vi "Sender 12 new version.vi"   [LabVIEW 2012]
uses:
  <vilib>/NXT/Block Support/NXT_OutputPort.ctl
  <vilib>/NXT/Block Support/NXT_MessageMailbox.ctl
  <vilib>/NXT/Block Support/NXT_InputPort.ctl
  <vilib>/NXT/Dual Mode Library/Waits/Wait_Num.vi
  <vilib>/NXT/Dual Mode Library/Motors/Rotation.vi
  <vilib>/NXT/Dual Mode Library/Motors/ResetMotor.vi
  <vilib>/NXT/Dual Mode Library/BT/BlueTooth_Write_String.vi
  <vilib>/NXT/Dual Mode Library/Display/drawText.vi
types:
  T1 = typedef "LVHSConnector.ctl" = refnum<class "BrickReference.lvclass">
  T2 = typedef "NXT_InputPort.ctl" = u32
  T3 = typedef "NXT_MessageMailbox.ctl" = u8
  T4 = typedef "NXT_OutputPort.ctl" = u8
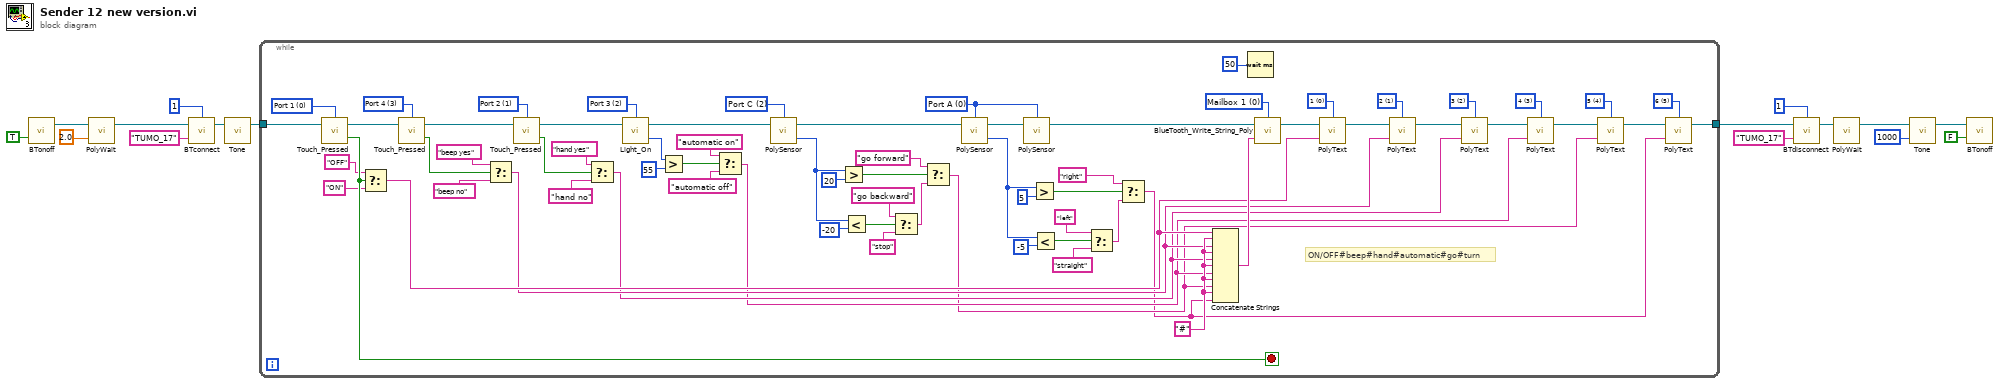
[diagram p0: block diagram]
diagram:
  n1 = call <vilib>:"BTonoff.vi"("On/Off"=TRUE) -> ("NXT/EV3"=w4:T1)  [unwired: 2 in, 1 out]
  n2 = call-poly <vilib>:"PolyWait.vi"("Time (1 sec)"=sgl 2.0, "NXT/EV3"=w4) -> ("NXT/EV3"=w3:T1)  [unwired: 2 in]
  n3 = call <vilib>:"BTconnect.vi"("Partner Name"="TUMO_17", "NXT/EV3"=w3, "Connection"=u8 1) -> ("NXT/EV3"=w10:T1)  [unwired: 1 out]
  n4 = call <vilib>:"Tone.vi"("NXT/EV3"=w10) -> ("NXT/EV3"=w9:T1)  [unwired: 3 in]
  n5 = while {
    tunnel: w9 -> [w67]
    tunnel: [w18] -> w1
    stop <- w66 stop-if-true
    w20 = i16 5 items=["1", "2", "3", "4", "5", "6", "7", "8", "9", "10", "11", "12"] ("Line")
    w23 = i16 4 items=["1", "2", "3", "4", "5", "6", "7", "8", "9", "10", "11", "12"] ("Line")
    w26 = i16 3 items=["1", "2", "3", "4", "5", "6", "7", "8", "9", "10", "11", "12"] ("Line")
    w29 = i16 2 items=["1", "2", "3", "4", "5", "6", "7", "8", "9", "10", "11", "12"] ("Line")
    w32 = i16 1 items=["1", "2", "3", "4", "5", "6", "7", "8", "9", "10", "11", "12"] ("Line")
    w34 = i16 0 items=["1", "2", "3", "4", "5", "6", "7", "8", "9", "10", "11", "12"] ("Line")
    w47 = T2 2 items=["Port 1", "Port 2", "Port 3", "Port 4"] ("Port (Port 1)")
    w55 = T2 1 items=["Port 1", "Port 2", "Port 3", "Port 4"] ("Port (Port 1)")
    w36 = "#" ("string")
    w69 = T2 0 items=["Port 1", "Port 2", "Port 3", "Port 4"] ("Port (Port 1)")
    w70 = u8 0 items=["Port A", "Port B", "Port C"] ("Port (Port A)")
    w78 = T2 3 items=["Port 1", "Port 2", "Port 3", "Port 4"] ("Port (Port 1)")
    w83 = T3 0 items=["Mailbox 1", "Mailbox 2", "Mailbox 3", "Mailbox 4", "Mailbox 5", "Mailbox 6", "Mailbox 7", "Mailbox 8", "Mailbox 9", "Mailbox 10"] ("Mailbox")
    w84 = T4 2 items=["Port A", "Port B", "Port C", "Port D"] ("Port (Port A)")
    # "ON/OFF#beep#hand#automatic#go#turn"
    n6 = call <vilib>:"Touch_Pressed.vi"("NXT/EV3"=w67, "Port (Port 1)"=w69) -> ("Yes / No"=w66:bool, "NXT/EV3"=w63:T1)  [unwired: 1 in]
    n7 = Select(t="OFF", s=w66, f="ON") -> (s? t:f=w33:string)
    n8 = call <vilib>:"Touch_Pressed.vi"("NXT/EV3"=w63, "Port (Port 1)"=w78) -> ("Yes / No"=w60:bool, "NXT/EV3"=w54:T1)  [unwired: 1 in]
    n9 = Select(t="beep yes", s=w60, f="beep no") -> (s? t:f=w30:string)
    n10 = call <vilib>:"Touch_Pressed.vi"("NXT/EV3"=w54, "Port (Port 1)"=w55) -> ("Yes / No"=w58:bool, "NXT/EV3"=w46:T1)  [unwired: 1 in]
    n11 = Select(t="hand yes", s=w58, f="hand no") -> (s? t:f=w27:string)
    n12 = call <vilib>:"Light_On.vi"("NXT/EV3"=w46, "Port (Port 3)"=w47) -> ("Scaled Value"=w45:i16, "NXT/EV3"=w42:T1)  [unwired: 1 in]
    n13 = Greater?(x=w45, y=i16 55) -> (0:w43:bool)
    n14 = Select(t="automatic on", s=w43, f="automatic off") -> (s? t:f=w24:string)
    n15 = call-poly <vilib>:"PolySensor.vi"("NXT/EV3"=w42, "Port (Port A)"=w84) -> ("Angle of Rotation"=w79:i32, "NXT/EV3"=w38:T1)  [unwired: 1 in]
    n16 = Greater?(x=w79, y=20) -> (0:w68:bool)
    n17 = Less?(x=w79, y=-20) -> (x < y?=w82:bool)
    n18 = Select(t="go backward", s=w82, f="stop") -> (s? t:f=w53:string)
    n19 = Select(t="go forward", s=w68, f=w53) -> (s? t:f=w21:string)
    n20 = call-poly <vilib>:"PolySensor.vi"("NXT/EV3"=w38, "Port (Port A)"=w70) -> ("Angle of Rotation"=w76:i32, "NXT/EV3"=w73:T1)  [unwired: 1 in]
    n21 = call-poly <vilib>:"PolySensor.vi"("NXT/EV3"=w73, "Port (All Ports)"=w70) -> ("NXT/EV3"=w37:T1)  [unwired: 2 in]
    n22 = Greater?(x=w76, y=5) -> (0:w74:bool)
    n23 = Less?(x=w76, y=-5) -> (x < y?=w72:bool)
    n24 = Select(t="left", s=w72, f="straight") -> (s? t:f=w71:string)
    n25 = Select(t="right", s=w74, f=w71) -> (s? t:f=w17:string)
    n26 = Concatenate Strings(w33, w36, w30, w36, w27, w36, w24, w36, w21, w36, w17) -> (w59:string)
    n27 = Wait (ms)(milliseconds to wait=u32 50) -> ()  [unwired: 1 out]
    n28 = call-poly <vilib>:"BlueTooth_Write_String_Poly.vi"("Message"=w59, "NXT/EV3"=w37, "Mailbox"=w83) -> ("NXT/EV3"=w35:T1)  [unwired: 1 in]
    n29 = call-poly <vilib>:"PolyText.vi"("Text"=w33, "NXT/EV3"=w35, "Line"=w34) -> ("NXT/EV3"=w31:T1)  [unwired: 1 in]
    n30 = call-poly <vilib>:"PolyText.vi"("Text"=w30, "NXT/EV3"=w31, "Line"=w32) -> ("NXT/EV3"=w28:T1)  [unwired: 1 in]
    n31 = call-poly <vilib>:"PolyText.vi"("Text"=w27, "NXT/EV3"=w28, "Line"=w29) -> ("NXT/EV3"=w25:T1)  [unwired: 1 in]
    n32 = call-poly <vilib>:"PolyText.vi"("Text"=w24, "NXT/EV3"=w25, "Line"=w26) -> ("NXT/EV3"=w22:T1)  [unwired: 1 in]
    n33 = call-poly <vilib>:"PolyText.vi"("Text"=w21, "NXT/EV3"=w22, "Line"=w23) -> ("NXT/EV3"=w19:T1)  [unwired: 1 in]
    n34 = call-poly <vilib>:"PolyText.vi"("Text"=w17, "NXT/EV3"=w19, "Line"=w20) -> ("NXT/EV3"=w18:T1)  [unwired: 1 in]
  }
  n35 = call <vilib>:"BTdisconnect.vi"("Partner Name"="TUMO_17", "NXT/EV3"=w1, "Connection"=u8 1) -> ("NXT/EV3"=w6:T1)  [unwired: 1 out]
  n36 = call-poly <vilib>:"PolyWait.vi"("NXT/EV3"=w6) -> ("NXT/EV3"=w5:T1)  [unwired: 3 in]
  n37 = call <vilib>:"Tone.vi"("Duration (500 ms)"=u16 1000, "NXT/EV3"=w5) -> ("NXT/EV3"=w8:T1)  [unwired: 2 in]
  n38 = call <vilib>:"BTonoff.vi"("On/Off"=FALSE, "NXT/EV3"=w8) -> ()  [unwired: 1 in, 2 out]
